vi "BrokerGetIOBuffer.vi"(9 "BufferKind":enum32{"Sent", "Received"}(ring)=enum."Received", 10 "DeviceID":u8=1, 11 "Handle In":u64[](array[numeric])) -> (1 "UsrData":u8[](array[numeric]), 2 "DataSize":i32, 3 "Handle Out":u64[](array[numeric]))   [LabVIEW 2020, in "SnapMB.lvlib"]
uses:
  SnapMB.lvlib
  windows/snapmb.dll
panel:
  out "error out":errorcluster
  in  "error in (no error)":errorcluster
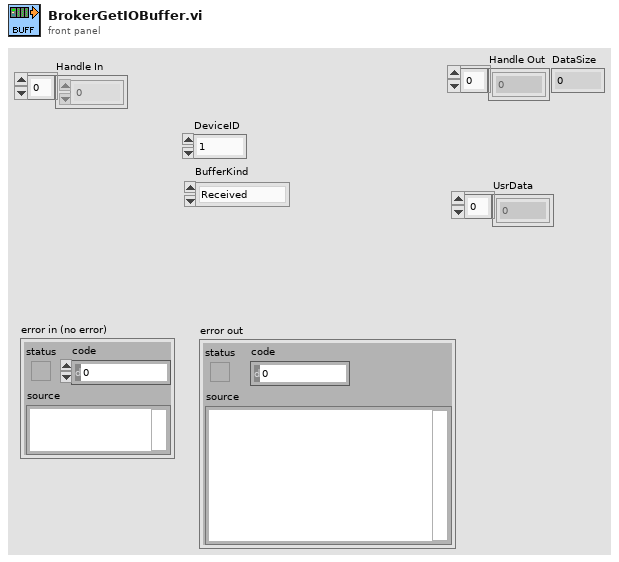
[diagram p1: front panel]
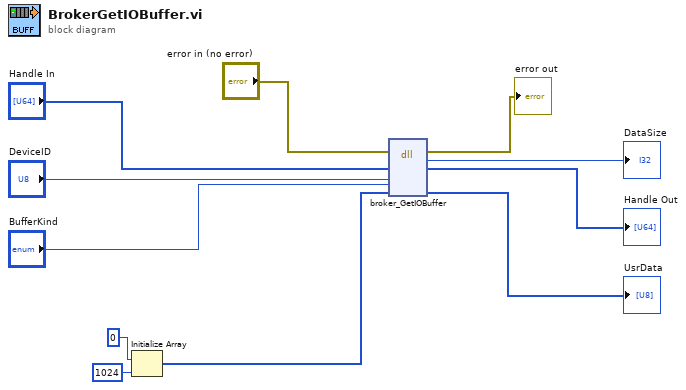
[diagram p0: block diagram]
diagram:
  n1 = Initialize Array(u8 0 ("element"), 1024 ("dimension size")) -> (w10:u8[])
  n2 = dll-call lib="D:/SnapMB/LabView/lib/windows/snapmb.dll" fn="broker_GetIOBuffer"(error in="error in (no error)", "Broker"="Handle In", "DeviceID"="DeviceID", "BufferKind"="BufferKind", "pUsrData"=w10) -> (error out=→"error out":errorcluster, "return type"=→"DataSize":i32, "Broker"=→"Handle Out":u64[], "pUsrData"=→"UsrData":u8[])  [unwired: 4 in, 1 out]
